vi "TankDrive.vi"(10 "right":dbl, 11 "left":dbl) -> ()   [LabVIEW 2015]
uses:
  <vilib>/Rock Robotics/WPI/Utilities/WPI_GetSetVariantRefNum.vi
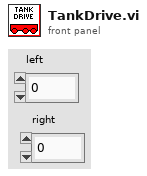
[diagram p1: front panel]
types:
  T1 = typedef "WPI_RobotDriveDevRef.ctl" = cluster{"DevStatus":errorcluster, "Motors[]":T2[], "Square Inputs":bool, "Max Output":dbl}
  T2 = typedef "WPI_MotorControlDeviceRef.ctl" = cluster{"DeviceStatus":errorcluster, "Type":T3, "PWM":cluster{"PWM Channel":T4, "DeadBand":T5}, "CAN":cluster{"Device Number":u8, "Control Mode":T6, "Semaphore":T7, "Max Vout":dbl, "TalonSRX Control Mode":T8}, "Invert":bool}
  T3 = typedef "WPI_MotorControlType.ctl" = enum16{"PWM", "CAN", "CANTalonSRX"}
  T4 = typedef "FPGA_DIOPWMChannel.ctl" = enum8{"PWM 0", "PWM 1", "PWM 2", "PWM 3", "PWM 4", "PWM 5", "PWM 6", "PWM 7", "PWM 8", "PWM 9", "PWM MXP 0", "PWM MXP 1", "PWM MXP 2", "PWM MXP 3", "PWM MXP 4", "PWM MXP 5", "PWM MXP 6", "PWM MXP 7", "PWM MXP 8", "PWM MXP 9", "Invalid"}
  T5 = typedef "WPI_PWMDeadband.ctl" = cluster{"Name":string, "maxPositivePwm":i32, "minPositivePwm":i32, "centerPwm":i32, "maxNegativePwm":i32, "minNegativePwm":i32, "angularRange":u16}
  T6 = typedef "WPI_CANJaguar_ControlMode.ctl" = enum8{"Percent VBus", "Current", "Speed", "Position", "Voltage"}
  T7 = typedef "Semaphore RefNum" = refnum<k1>
  T8 = typedef "WPI_CANTalonSRX_APIControlMode.ctl" = enum8{"Percent VBus", "Speed", "Position", "Slave", "Unchanged / Invalid", "Voltage Compensation", "Current", "Motion Profile"}
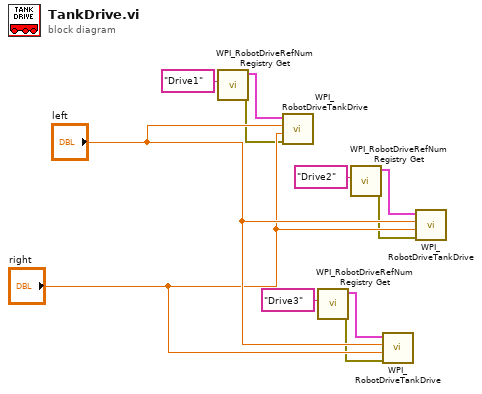
[diagram p0: block diagram]
diagram:
  n1 = call <vilib>:"WPI_RobotDriveRefNum Registry Get.vi"("refnum name"="Drive1") -> ("error out"=w7:errorcluster, "RobotDriveDevRef"=w8:T1)  [unwired: 9 in]
  n2 = call <vilib>:"WPI_RobotDriveTankDrive.vi"("error in (no error)"=w7, "Right axis value"="right", "Left axis value"="left", "RobotDriveDevRef"=w8) -> ()  [unwired: 5 in, 3 out]
  n3 = call <vilib>:"WPI_RobotDriveRefNum Registry Get.vi"("refnum name"="Drive3") -> ("error out"=w1:errorcluster, "RobotDriveDevRef"=w2:T1)  [unwired: 9 in]
  n4 = call <vilib>:"WPI_RobotDriveRefNum Registry Get.vi"("refnum name"="Drive2") -> ("error out"=w4:errorcluster, "RobotDriveDevRef"=w5:T1)  [unwired: 9 in]
  n5 = call <vilib>:"WPI_RobotDriveTankDrive.vi"("error in (no error)"=w1, "Right axis value"="right", "Left axis value"="left", "RobotDriveDevRef"=w2) -> ()  [unwired: 5 in, 3 out]
  n6 = call <vilib>:"WPI_RobotDriveTankDrive.vi"("error in (no error)"=w4, "Right axis value"="right", "Left axis value"="left", "RobotDriveDevRef"=w5) -> ()  [unwired: 5 in, 3 out]
